vi "Fix Precision.vi"(11 "DBL":dbl[](array[numeric])) -> (3 "DBLOut":dbl[](array[numeric]))   [LabVIEW 2011]
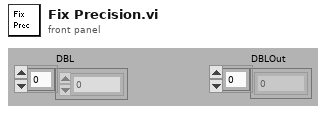
[diagram p1: front panel]
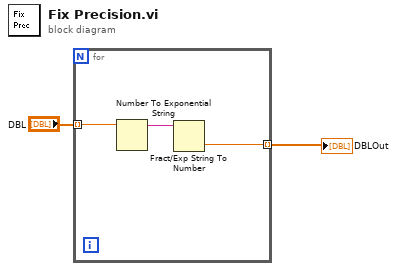
[diagram p0: block diagram]
diagram:
  n1 = for {
    tunnel: "DBL" -> [w5] mode=indexing
    tunnel: [w3] -> w1 mode=indexing
    n2 = Number To Exponential String(number=w5) -> (E-format string=w4:string)  [unwired: 3 out]
    n3 = Fract/Exp String To Number(string=w4) -> (number=w3:dbl)  [unwired: 4 out]
  }
  "DBLOut" <- w1
